vi "Parse Packet.vi"(11 "Packet":string) -> (3 "Packet Data":T1[](array[typedef]))   [LabVIEW 2022 SP3, in "AoC22.lvlib"]
uses:
  AoC22.lvlib
  Packet Item.ctl
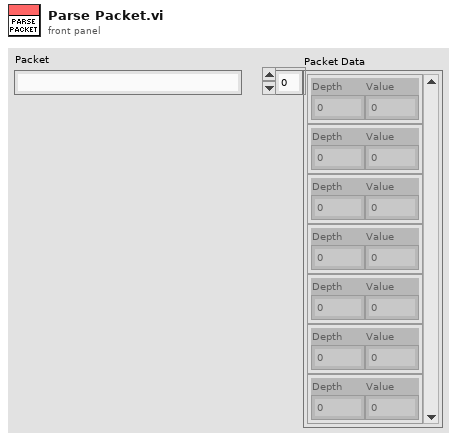
[diagram p1: front panel]
types:
  T1 = typedef "AoC22.lvlib/Packet Item.ctl" = cluster{"Depth":i32, "Value":i32}
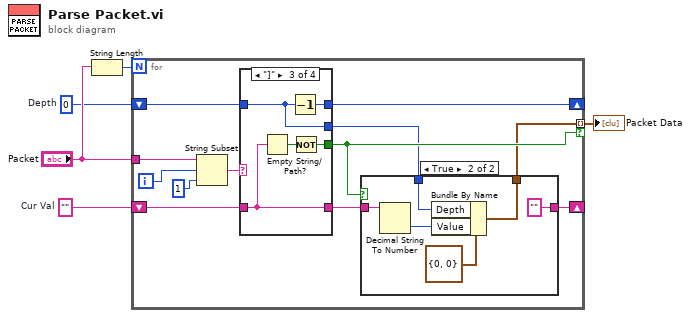
[diagram p0: block diagram]
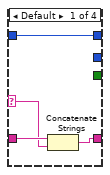
[diagram p2: hidden frame]
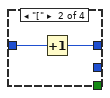
[diagram p3: hidden frame]
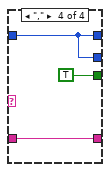
[diagram p4: hidden frame]
diagram:
  w2 = ""  # Cur Val
  w3 = 0  # Depth
  n1 = String Length(string="Packet") -> (length=w5:i32)
  n2 = for {
    N: w5 -> [_]
    tunnel: "Packet" -> [w17]
    shift-right: [w9] -> _
    shift-left: w3 -> [w12]
    shift-right: [w8] -> _
    shift-left: w2 -> [w13]
    tunnel: [w7] -> w1 mode=indexing if=w10
    i -> [w16]
    n3 = String Subset(string=w17, offset (0)=w16, length (rest)=1 ("length (rest)")) -> (substring=w14:string)
    n4 = case shown="\"]\"" w14 {
      selector: w14 -> [w20 _ _ _]
      tunnel: w13 -> [w21 _ w26 w30]
      tunnel: w12 -> [w18 w23 w27 w29]
      tunnel: [w18 w22 w28 w29] -> w9
      tunnel: [_ _ w25 TRUE] -> w10
      tunnel: [w19 _ w26 w30] -> w11
      tunnel: [_ _ w27 w29] -> w6
      frame Default {
        n5 = Concatenate Strings(w21, w20) -> (w19:string)
      }
      frame "[" {
        n6 = Increment(x=w23) -> (x+1=w22:i32)
      }
      frame "]" {
        n7 = Empty String/Path?(string/path=w26) -> (empty?=w24:bool)
        n8 = Decrement(x=w27) -> (x-1=w28:i32)
        n9 = Not(x=w24) -> (.not. x?=w25:bool)
      }
      frame "," {
      }
    }
    n10 = case shown="True" w10 {
      tunnel: w11 -> [w32 w38]
      tunnel: w6 -> [_ w35]
      tunnel: [w32 "" ("Cur Val")] -> w8
      tunnel: [_ w34] -> w7
      frame False {
      }
      frame True {
        n11 = Decimal String To Number(string=w38) -> (number=w36:i32)  [unwired: 2 in, 1 out]
        n12 = Bundle By Name(cluster=T1 {"Depth"=0, "Value"=0} ("Packet Item"), "Depth"=w35, "Value"=w36) -> (w34:T1)
      }
    }
  }
  "Packet Data" <- w1
